vi "GraphLockin_vs_Parameter.vi"(4 "V-":i32=1 min=1, 6 "V+":i32=1 min=1, 7 "reset?":bool, 8 "Current":i32=1 min=1, 9 "Parameter":dbl, 10 "Y[ ]":dbl[](array[numeric]), 11 "X[ ]":dbl[](array[numeric])) -> (0 "R(Ohms) vs Parameter":cluster{"Y":dbl[], "Y":dbl[]}[](graph), 1 "G(e2/h) vs Parameter":cluster{"Y":dbl[], "Y":dbl[]}[](graph), 2 "Y vs Parameter":cluster{dbl[], dbl[]}[](graph), 3 "X vs Parameter":cluster{dbl[], dbl[]}[](graph))   [LabVIEW 2019, in "SMO.Transport.lvclass"]
uses:
  SMO.Transport.lvclass
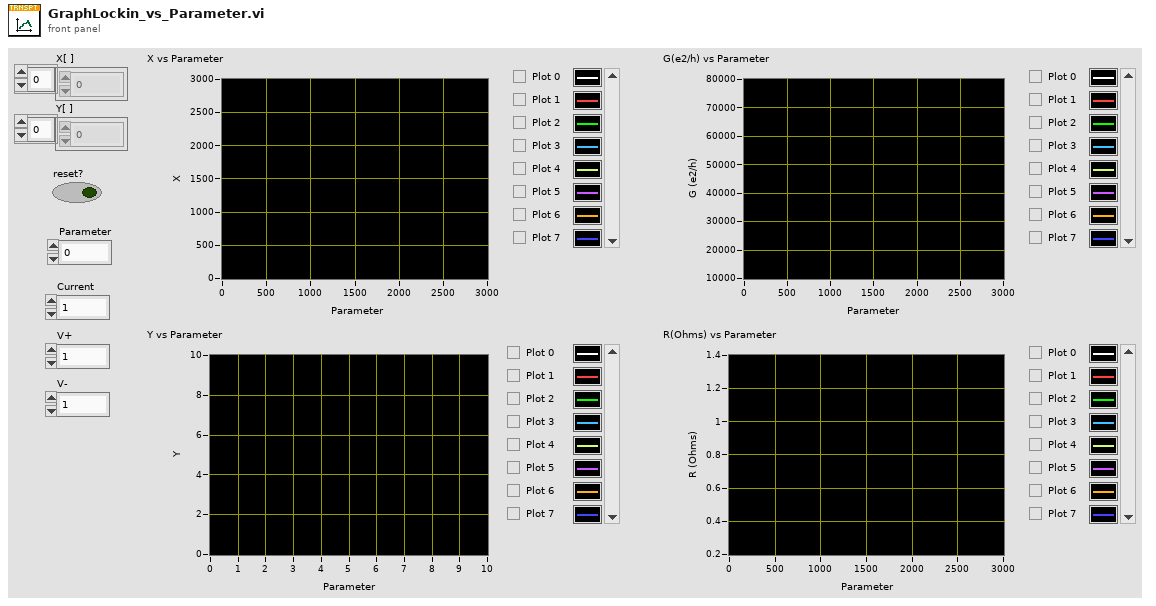
[diagram p1: front panel]
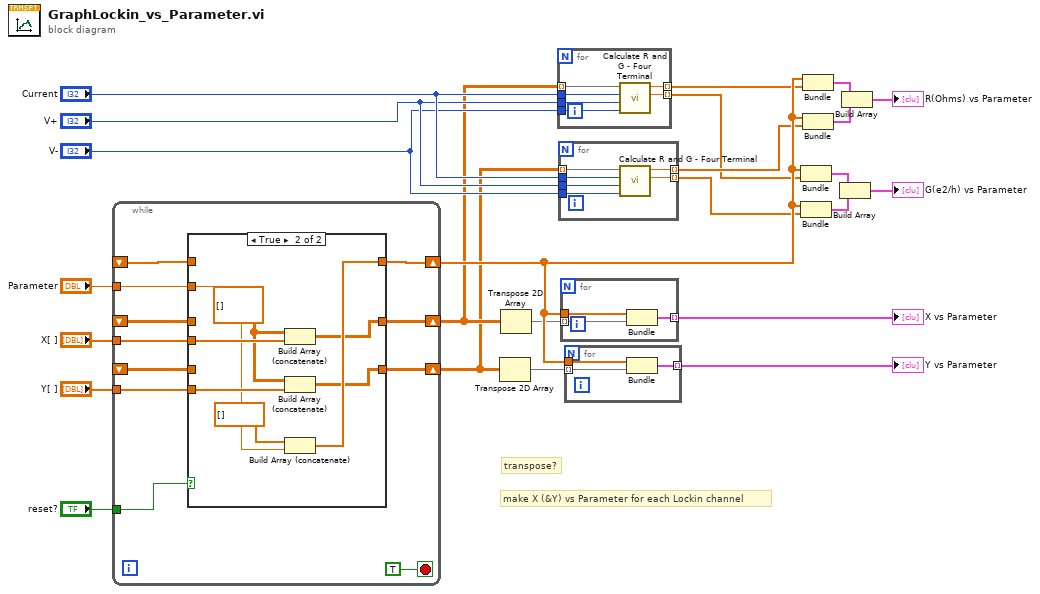
[diagram p0: block diagram]
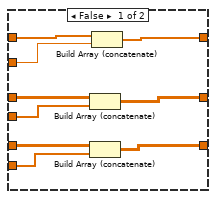
[diagram p2: hidden frame]
diagram:
  # "make X (&Y) vs Parameter for each Lockin channel"
  # "transpose?"
  n1 = while {
    tunnel: "X[ ]" -> [w35]
    tunnel: "Parameter" -> [w34]
    tunnel: "reset?" -> [w32]
    shift-right: [w25] -> w2
    shift-left: _ -> [w31]
    shift-right: [w26] -> w1
    shift-left: _ -> [w29]
    tunnel: "Y[ ]" -> [w30]
    shift-right: [w27] -> w13
    shift-left: _ -> [w28]
    stop <- TRUE stop-if-true
    n2 = case shown="True" w32 {
      tunnel: w35 -> [w44 w52]
      tunnel: w34 -> [w39 w48]
      tunnel: [w36 w46] -> w25
      tunnel: w31 -> [w43 _]
      tunnel: w30 -> [w42 w50]
      tunnel: w29 -> [w41 _]
      tunnel: [w37 w45] -> w26
      tunnel: [w38 w47] -> w27
      tunnel: w28 -> [w40 _]
      frame False {
        n3 = Build Array (concatenate)(w43, w44) -> (w36:dbl[][])
        n4 = Build Array (concatenate)(w41, w42) -> (w37:dbl[][])
        n5 = Build Array (concatenate)(w40, w39) -> (w38:dbl[])
      }
      frame True {
        w51 = dbl[][] []
        n6 = Build Array (concatenate)(w51, w52) -> (w46:dbl[][])
        n7 = Build Array (concatenate)(w51, w50) -> (w45:dbl[][])
        n8 = Build Array (concatenate)(dbl[] [], w48) -> (w47:dbl[])
      }
    }
  }
  n9 = Transpose 2D Array(2D array=w1) -> (transposed array=w3:dbl[][])
  n10 = Transpose 2D Array(2D array=w2) -> (transposed array=w4:dbl[][])
  n11 = for {
    tunnel: "Current" -> [w58]
    tunnel: "V+" -> [w57]
    tunnel: "V-" -> [w56]
    tunnel: [w55] -> w8 mode=indexing
    tunnel: [w54] -> w6 mode=indexing
    tunnel: w2 -> [w53] mode=indexing
    n12 = call "Calculate R and G - Four Terminal.vi"("V-"=w56, "V+"=w57, "Current"=w58, "Lockin[ ]"=w53) -> ("G_4T (e2/h)"=w54:dbl, "R_4T (ohms)"=w55:dbl)  [unwired: 6 in]
  }
  n13 = for {
    tunnel: "Current" -> [w64]
    tunnel: "V+" -> [w63]
    tunnel: "V-" -> [w62]
    tunnel: [w61] -> w7 mode=indexing
    tunnel: [w60] -> w5 mode=indexing
    tunnel: w1 -> [w59] mode=indexing
    n14 = call "Calculate R and G - Four Terminal.vi"("V-"=w62, "V+"=w63, "Current"=w64, "Lockin[ ]"=w59) -> ("G_4T (e2/h)"=w60:dbl, "R_4T (ohms)"=w61:dbl)  [unwired: 6 in]
  }
  n15 = for {
    tunnel: [w67] -> w20 mode=indexing
    tunnel: w13 -> [w66]
    tunnel: w4 -> [w65] mode=indexing
    n16 = Bundle(w66, w65) -> (w67:cluster{dbl[], dbl[]})  [unwired: 1 in]
  }
  "X vs Parameter" <- w20
  n17 = for {
    tunnel: [w70] -> w19 mode=indexing
    tunnel: w13 -> [w69]
    tunnel: w3 -> [w68] mode=indexing
    n18 = Bundle(w69, w68) -> (w70:cluster{dbl[], dbl[]})  [unwired: 1 in]
  }
  "Y vs Parameter" <- w19
  n19 = Bundle(w13, w6) -> (w18:cluster{dbl[], dbl[]})  [unwired: 1 in]
  n20 = Bundle(w13, w5) -> (w16:cluster{dbl[], dbl[]})  [unwired: 1 in]
  n21 = Bundle(w13, w8) -> (w14:cluster{dbl[], dbl[]})  [unwired: 1 in]
  n22 = Bundle(w13, w7) -> (w15:cluster{dbl[], dbl[]})  [unwired: 1 in]
  n23 = Build Array(w18, w16) -> (→"G(e2/h) vs Parameter":cluster{dbl[], dbl[]}[])
  n24 = Build Array(w14, w15) -> (→"R(Ohms) vs Parameter":cluster{dbl[], dbl[]}[])
